vi "Get Observables for Quality Check.vi"(8 "error in (no error)":errorcluster, 11 "Monkey in":refnum<class "Monkey.lvclass">=refnum) -> (0 "error out":errorcluster, 2 "Obsv to check":T1(array[cluster]), 3 "Monkey out":refnum<class "Monkey.lvclass">)   [LabVIEW 2020, in "CIRCUS_uServices.lvlib" / "Holy Trinity.lvlib" / "Monkey.lvlib" / "Monkey.lvclass"]
uses:
  Monkey.lvclass
  Run Utilities/Run Block/Run Block.lvclass
  Run Utilities/Run Instance/Run Instance.lvclass
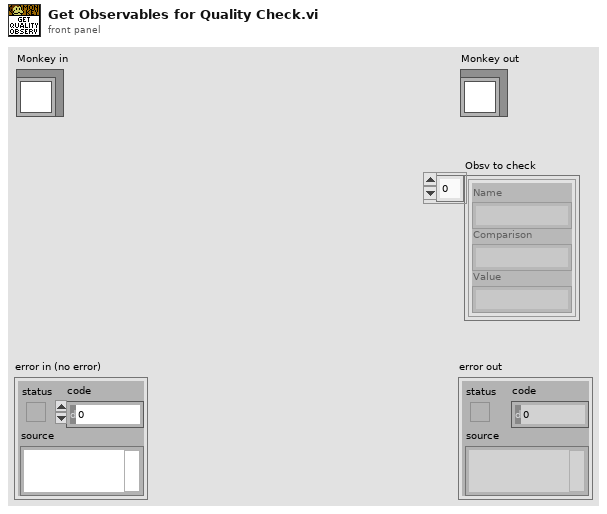
[diagram p1: front panel]
types:
  T1 = cluster{"Name":string, "Comparison":string, "Value":string}[]
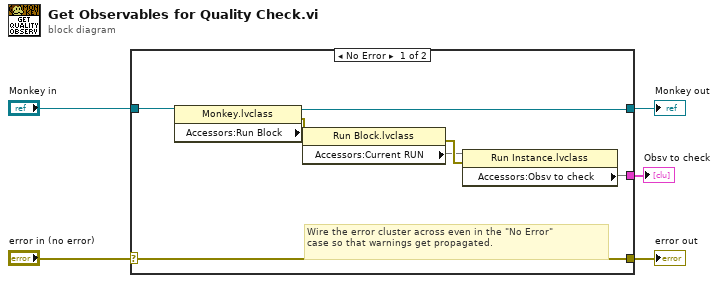
[diagram p0: block diagram]
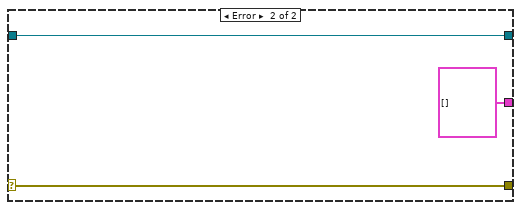
[diagram p2: hidden frame]
diagram:
  n1 = case shown="No Error" "error in (no error)" {
    selector: "error in (no error)" -> [w12 w16]
    tunnel: [w12 w16] -> w4
    tunnel: [w9 w15] -> w2
    tunnel: "Monkey in" -> [w10 w15]
    tunnel: [w6 T1 [] ("Accessors:Obsv to check")] -> w1
    frame No Error {
      # "Wire the error cluster across even in the \"No Error\"\ncase so that warnings get propagated."
      n2 = property class="Monkey.lvclass"(reference=w10) -> (reference out=w9:refnum<class "Monkey.lvclass">, error out=w13:errorcluster, "Accessors:Run Block"=w11)  [unwired: 1 in]
      n3 = property class="Run Block.lvclass"(reference=w11, error in=w13) -> (error out=w8:errorcluster, "Accessors:Current RUN"=w7)  [unwired: 1 out]
      n4 = property class="Run Instance.lvclass"(reference=w7, error in=w8) -> ("Accessors:Obsv to check"=w6)  [unwired: 2 out]
    }
    frame Error {
    }
  }
  "error out" <- w4
  "Monkey out" <- w2
  "Obsv to check" <- w1
